vi "Terminal Type Matches Patterns.vi"(5 "Enum Names ?":bool, 7 "Include Names":bool, 8 "error in (no error)":errorcluster, 10 "Terminal Type patterns List":string[](array[string]), 11 "Terminal":T1) -> (0 "error out":errorcluster, 1 "Which Pattern matches ?":i32, 3 "Terminal Matches Pattern ?":bool)   [LabVIEW 2018, in "Scripting Tools.lvlib" / "XNode Support.lvlib"]
doc: "Tests whether ther data type for <b>Terminal</b> has a string representation that matches one of a list of regular expression patterns <b>Terminal Type Patterns List</b> and if so, which one . The options <b>Include Names</b> and <b>Enum names ?</b> are used to determine whether the type representations tring includes element names and enum labels."
uses:
  XNode Support.lvlib
  <vilib>/XNodeSupport/XNodeTermIDPair.ctl
  <vilib>/XNodeSupport/XNodeTermRef.ctl
  <vilib>/XNodeSupport/XNodeString.ctl
  <vilib>/XNodeSupport/NI_XNodeSupport.lvlib
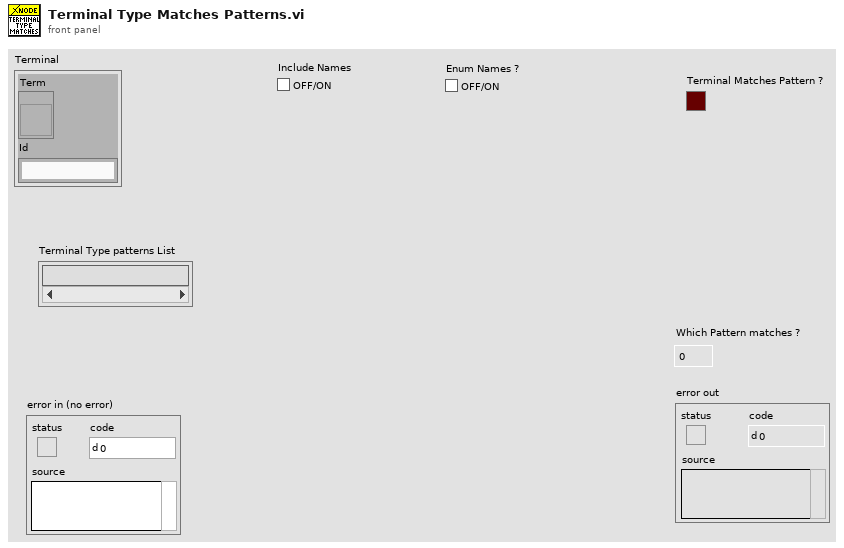
[diagram p1: front panel]
types:
  T1 = typedef "NI_XNodeSupport.lvlib/XNodeTermIDPair.ctl" = cluster{"Term":T2, "Id":T3}
  T2 = typedef "NI_XNodeSupport.lvlib/XNodeTermRef.ctl" = refnum<vi>
  T3 = typedef "NI_XNodeSupport.lvlib/XNodeString.ctl" = string
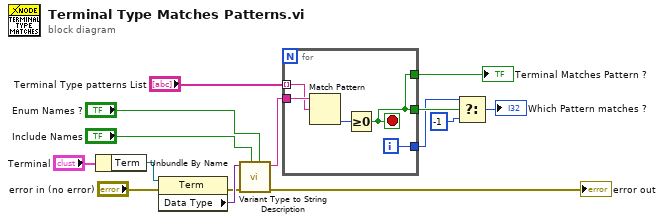
[diagram p0: block diagram]
diagram:
  n1 = Unbundle By Name("Terminal") -> ("Term"=w14:T2)
  n2 = property class="Term"(reference=w14, error in="error in (no error)") -> (error out=w12:errorcluster, "Data Type"=w13:variant)  [unwired: 1 out]
  n3 = call "Variant Type to String Description.vi"("Enum Names ?"="Enum Names ?", "Include Names"="Include Names", "error in (no error)"=w12, "Data Type"=w13) -> ("error out"=→"error out":errorcluster, "String Representation of Type"=w8:string)  [unwired: 5 in, 1 out]
  n4 = for {
    tunnel: w8 -> [w20]
    tunnel: [w17] -> w6
    tunnel: "Terminal Type patterns List" -> [w18] mode=indexing
    tunnel: [w17] -> w4
    tunnel: [w16] -> w3
    i -> [w16]
    stop <- w17 stop-if-true
    n5 = Match Pattern(string=w20, regular expression=w18) -> (offset past match=w19:i32)  [unwired: 1 in, 3 out]
    n6 = Greater Or Equal To 0?(x=w19) -> (x >= 0?=w17:bool)
  }
  "Terminal Matches Pattern ?" <- w6
  n7 = Select(t=w3, s=w4, f=-1) -> (s? t:f=→"Which Pattern matches ?":i32)
